vi "Unmarshal.vi"(8 "error in (no error)":errorcluster, 10 "Buffer":u8[](array[numeric]), 11 "int32 in":refnum<class "fixed32.lvclass">) -> (0 "error out":errorcluster, 2 "Buffer Count":i32, 3 "int32 out":refnum<class "fixed32.lvclass">)   [LabVIEW 2020, in "Protobuf RAW.lvlib" / "fixed32.lvclass"]
uses:
  fixed32.lvclass
  fixed32.lvclass/fixed32.ctl
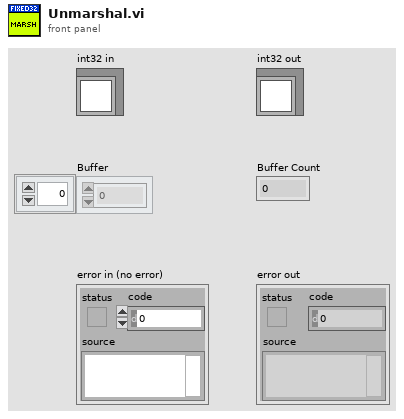
[diagram p1: front panel]
types:
  T1 = enum16{"big-endian, network order", "native, host order", "little-endian"}
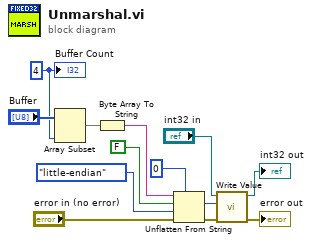
[diagram p0: block diagram]
diagram:
  w9 = 4 ("index")
  n1 = Array Subset(array="Buffer", length=w9) -> (w10:u8[])  [unwired: 1 in]
  n2 = Byte Array To String(unsigned byte array=w10) -> (string=w3:string)
  n3 = Unflatten From String(type=u32 0 ("Value"), binary string=w3, data includes array or string size? (T)=FALSE, byte order (0:big-endian, network order)=T1."little-endian", error in (no error)="error in (no error)") -> (value=w6:u32, error out=w12:errorcluster)  [unwired: 1 out]
  n4 = call "Write Value.vi"("error in (no error)"=w12, "Value"=w6, "fixed32 in"="int32 in") -> ("error out"=→"error out":errorcluster, "fixed32 out"=→"int32 out":refnum<class "fixed32.lvclass">)  [unwired: 7 in]
  "Buffer Count" <- w9
